vi "WD_update_barcode.vi"(5 "NULL: workplace_id":i16=-1, 7 "Set null":bool=TRUE, 8 "error in (no error)":errorcluster, 9 "Workplace data":cluster{"barcode A":string, "barcode B":string}={"barcode A"="509", "barcode B"="123"}, 10 "workplace_id":i16=5, 11 "DBlink":string="Driver={ODBC Driver 17 for SQL Server};Server=localhost\\SQLEXPRESS;Database=ZDX201;UID=labview;PWD=Dsa@54137926") -> ()   [LabVIEW 2019]
uses:
  <vilib>/addons/database/Connection.llb/DB Tools Open Connec (String).vi
  <vilib>/addons/database/Connection.llb/Conn Execute.vi
  <vilib>/addons/database/Recordset.llb/Rec Fetch Recordset Data (R).vi
  <vilib>/addons/database/Recordset.llb/Rec Destroy - Connection.vi
  <vilib>/addons/database/_DB Variant To Data/Database Variant To Data.xnode
  <vilib>/addons/database/NI_Database_API.lvlib
panel:
  out "length":i32
  out "substring":string
  out "查詢結果":string="Update [workplace_data] \nset  \n[barcode A] = NULL       \n  ,[barcode B] = NULL\n \n  where [workplace_name_id]= -1"
  out "Workplace: assemble":cluster{"條碼A":string, "條碼B":string}[](array[cluster])
  out "Command":string="where [workplace_name_id]= 5"
  out "update value":T1={"barcode A"="509", "barcode B"="123", "update time"=timestamp(3738130170.8632746 s since 1904-01-01)} {"update time" format="%<%.0X %x>T"}
  in  "columns":string[](array[string])=["[barcode A]", "[barcode B]", "update_time"]
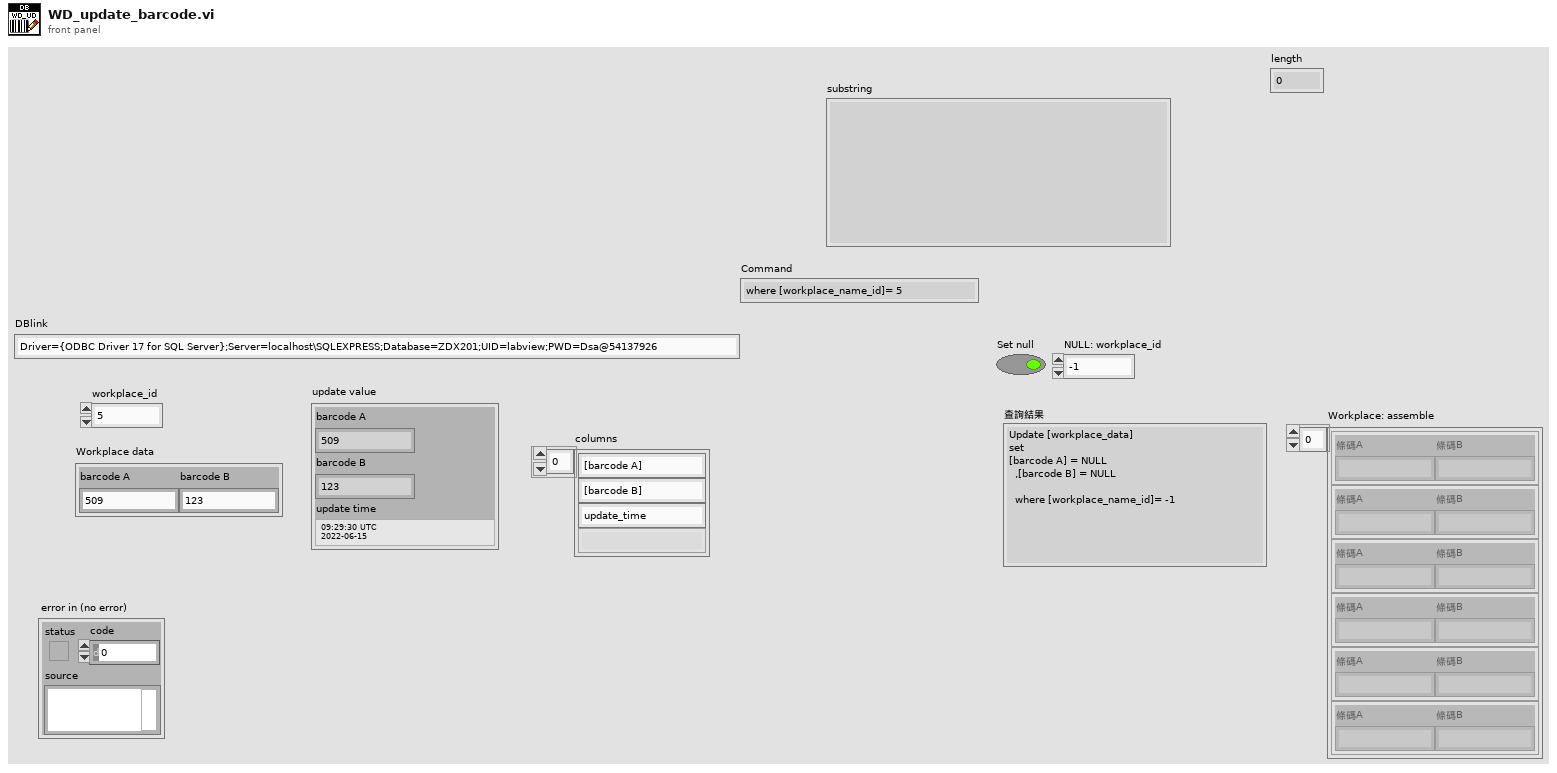
[diagram p1: front panel]
types:
  T1 = cluster{"barcode A":string, "barcode B":string, "update time":timestamp}
  T2 = typedef "NI_Database_API.lvlib/Conn ObjectReference.ctl" = refnum<k1>
  T3 = typedef "NI_Database_API.lvlib/Rec ObjectReference.ctl" = refnum<k1>
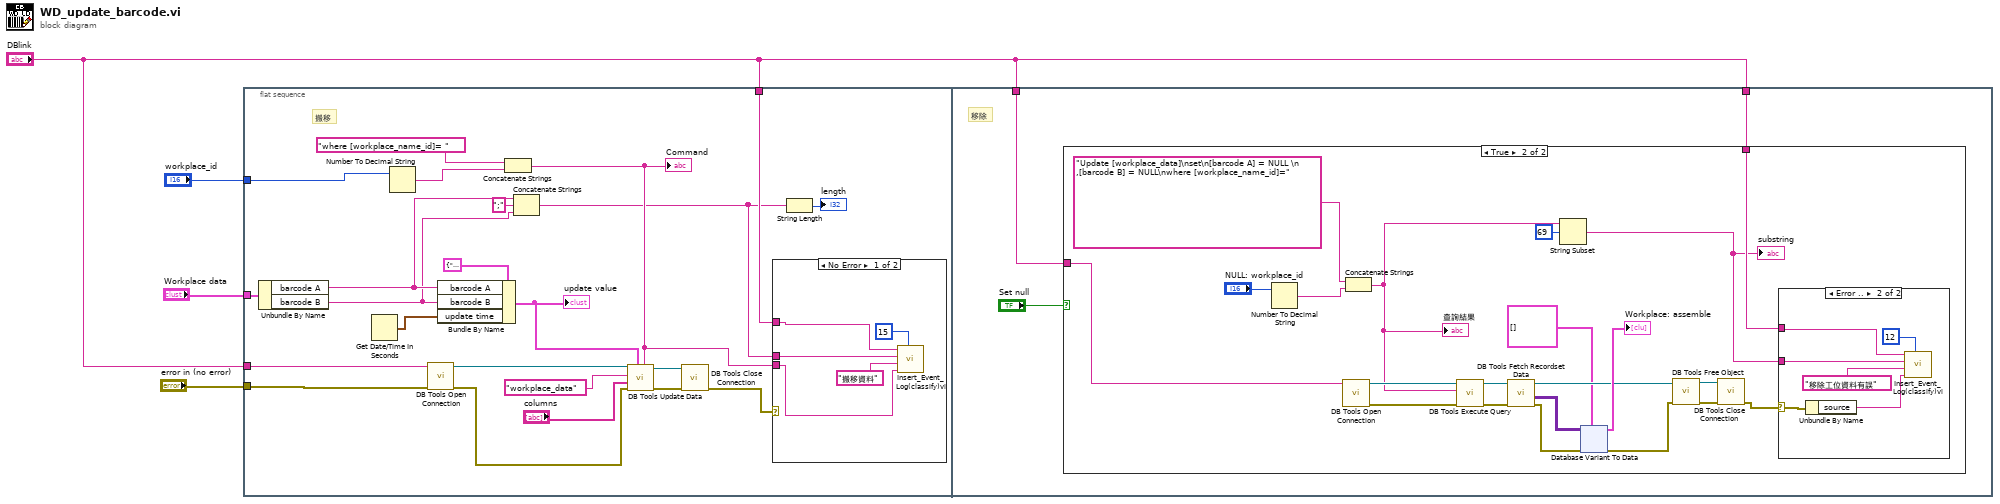
[diagram p0: block diagram]
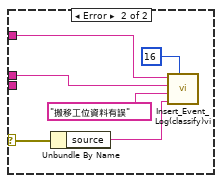
[diagram p2: hidden frame]
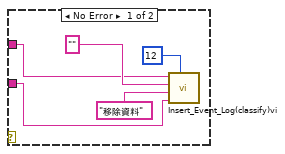
[diagram p4: hidden frame]
diagram:
  n1 = flat-sequence {
    tunnel: "error in (no error)" -> [w27]
    tunnel: "workplace_id" -> [w20]
    tunnel: "Workplace data" -> [w14]
    tunnel: "DBlink" -> [w13]
    tunnel: "DBlink" -> [w11]
    tunnel: "DBlink" -> [w40]
    tunnel: "DBlink" -> [w39]
    frame #0 {
      # "搬移"
      n2 = Unbundle By Name(w14) -> ("barcode A"=w9:string, "barcode B"=w7:string)
      n3 = Get Date/Time In Seconds() -> (seconds since 1Jan1904=w19:timestamp)
      n4 = Number To Decimal String(number=w20) -> (decimal integer string=w17:string)  [unwired: 1 in]
      n5 = call-poly <vilib>:"DB Tools Open Connection.vi"("error in (no error)"=w27, "connection information"=w13) -> ("error out"=w25:errorcluster, "connection reference"=w23:T2)  [unwired: 6 in]
      n6 = Bundle By Name(cluster=T1 {"barcode A"="", "barcode B"="", "update time"=timestamp(0 s since 1904-01-01)} ("update value"), "barcode A"=w9, "barcode B"=w7, "update time"=w19) -> (w15:T1)
      "update value" <- w15
      n7 = Concatenate Strings("where [workplace_name_id]= ", w17) -> (w10:string)
      "Command" <- w10
      n8 = Concatenate Strings(w9, ";" ("string"), w7) -> (w6:string)
      n9 = call <vilib>:"DB Tools Update Data.vi"("condition"=w10, "data"=w15, "error in (no error)"=w25, "columns"="columns", "table"="workplace_data", "connection reference"=w23) -> ("error out"=w26:errorcluster, "connection reference out"=w24:T2)  [unwired: 4 in]
      n10 = call <vilib>:"DB Tools Close Connection.vi"("error in (no error)"=w26, "connection reference"=w24) -> ("error out"=w12:errorcluster)  [unwired: 5 in]
      n11 = case shown="No Error" w12 {
        selector: w12 -> [_ w35]
        tunnel: w11 -> [w30 w38]
        tunnel: w10 -> [w29 _]
        tunnel: w6 -> [w28 w33]
        frame No Error {
          n12 = call "Insert_Event_Log(classify)vi.vi"("classify"=i16 15, "data"=w29, "message"="搬移資料", "id"=w28, "DBlink"=w30) -> ()  [unwired: 6 in, 1 out]
        }
        frame Error {
          n13 = Unbundle By Name(w35) -> ("source"=w34:string)
          n14 = call "Insert_Event_Log(classify)vi.vi"("classify"=i16 16, "data"=w34, "message"="搬移工位資料有誤", "id"=w33, "DBlink"=w38) -> ()  [unwired: 6 in, 1 out]
        }
      }
      n15 = String Length(string=w6) -> (length=→"length":i32)
    }
    frame #1 {
      # "移除"
      n16 = case shown="True" "Set null" {
        tunnel: w40 -> [_ w48]
        tunnel: w39 -> [_ w47]
        frame False {
        }
        frame True {
          n17 = Number To Decimal String(number="NULL: workplace_id") -> (decimal integer string=w46:string)  [unwired: 1 in]
          n18 = call-poly <vilib>:"DB Tools Open Connection.vi"("connection information"=w48) -> ("error out"=w51:errorcluster, "connection reference"=w52:T2)  [unwired: 7 in]
          n19 = Concatenate Strings("Update [workplace_data]\nset\n[barcode A] = NULL \n ,[barcode B] = NULL\nwhere [workplace_name_id]=", w46) -> (w44:string)
          "查詢結果" <- w44
          n20 = call-poly <vilib>:"DB Tools Execute Query.vi"("error in (no error)"=w51, "SQL query"=w44, "connection reference"=w52) -> ("error out"=w54:errorcluster, "recordset reference"=w53:T3)  [unwired: 5 in]
          n21 = call-poly <vilib>:"DB Tools Fetch Recordset Data.vi"("error in (no error)"=w54, "recordset reference"=w53) -> ("error out"=w59:errorcluster, "recordset data"=w60:variant[][], "recordset reference out"=w58:T3)  [unwired: 3 in]
          n22 = String Subset(string=w44, offset (0)=69) -> (substring=w42:string)  [unwired: 1 in]
          "substring" <- w42
          n23 = xnode "Database Variant To Data"("database variant"=w60, "error in (no error)"=w59, "type"=cluster{"條碼A":string, "條碼B":string}[] [] ("Workplace: assemble")) -> ("data"=→"Workplace: assemble":cluster{"條碼A":string, "條碼B":string}[], "error out"=w57:errorcluster)
          n24 = call-poly <vilib>:"DB Tools Free Object.vi"("error in (no error)"=w57, "recordset reference"=w58) -> ("error out"=w56:errorcluster, "connection reference"=w55:T2)  [unwired: 8 in]
          n25 = call <vilib>:"DB Tools Close Connection.vi"("error in (no error)"=w56, "connection reference"=w55) -> ("error out"=w45:errorcluster)  [unwired: 5 in]
          n26 = case shown="Error .." w45 {
            selector: w45 -> [_ w70]
            tunnel: w47 -> [w64 w73]
            tunnel: w42 -> [w63 w68]
            frame No Error {
              n27 = call "Insert_Event_Log(classify)vi.vi"("classify"=i16 12, "data"=w63, "message"="移除資料", "id"="", "DBlink"=w64) -> ()  [unwired: 6 in, 1 out]
            }
            frame Error {
              n28 = Unbundle By Name(w70) -> ("source"=w69:string)
              n29 = call "Insert_Event_Log(classify)vi.vi"("classify"=i16 12, "data"=w69, "message"="移除工位資料有誤", "id"=w68, "DBlink"=w73) -> ()  [unwired: 6 in, 1 out]
            }
          }
        }
      }
    }
  }
